vi "Playback Floor.vi"(0 "Encoder Names":string[](array[string])=["X axis", "Y axis"], 1 "Floor Recording Data":T2={"X Axis Recording Data"=[{"Encoder Position"=0.0, "Timestamp"=21}, {"Encoder Position"=0.0, "Timestamp"=41}, {"Encoder Position"=0.0, "Timestamp"=62}, {"Encoder Position"=0.0, "Timestamp"=82}, {"Encoder Position"=0.25, "Timestamp"=102}, {"Encoder Position"=0.25, "Timestamp"=122}, {"Encoder Position"=0.25, "Timestamp"=143}, {"Encoder Position"=0.25, "Timestamp"=162}, {"Encoder Position"=0.25, "Timestamp"=182}, {"Encoder Position"=0.25, "Timestamp"=202}, {"Encoder Position"=0.25, "Timestamp"=222}, {"Encoder Position"=0.75, "Timestamp"=242}, {"Encoder Position"=1.5, "Timestamp"=262}, {"Encoder Position"=2.25, "Timestamp"=282}, {"Encoder Position"=3.0, "Timestamp"=302}, {"Encoder Position"=3.75, "Timestamp"=323}, {"Encoder Position"=4.75, "Timestamp"=342}, {"Encoder Position"=5.25, "Timestamp"=363}, {"Encoder Position"=5.75, "Timestamp"=382}, {"Encoder Position"=6.5, "Timestamp"=402}, {"Encoder Position"=7.0, "Timestamp"=422}, {"Encoder Position"=7.5, "Timestamp"=443}, {"Encoder Position"=8.0, "Timestamp"=462}, {"Encoder Position"=8.25, "Timestamp"=482}, {"Encoder Position"=8.75, "Timestamp"=502}, {"Encoder Position"=8.75, "Timestamp"=522}, {"Encoder Position"=9.25, "Timestamp"=542}, {"Encoder Position"=9.25, "Timestamp"=562}, {"Encoder Position"=9.5, "Timestamp"=582}, {"Encoder Position"=9.75, "Timestamp"=602}, {"Encoder Position"=9.75, "Timestamp"=622}, {"Encoder Position"=9.75, "Timestamp"=642}, {"Encoder Position"=9.75, "Timestamp"=662}, {"Encoder Position"=9.75, "Timestamp"=683}, {"Encoder Position"=9.75, "Timestamp"=702}, {"Encoder Position"=9.75, "Timestamp"=722}, {"Encoder Position"=9.75, "Timestamp"=743}, {"Encoder Position"=10.0, "Timestamp"=763}, {"Encoder Position"=10.0, "Timestamp"=784}, {"Encoder Position"=10.25, "Timestamp"=803}, {"Encoder Position"=10.25, "Timestamp"=824}, {"Encoder Position"=10.75, "Timestamp"=844}, {"Encoder Position"=11.0, "Timestamp"=864}, {"Encoder Position"=11.5, "Timestamp"=884}, {"Encoder Position"=12.25, "Timestamp"=904}, {"Encoder Position"=13.25, "Timestamp"=924}, {"Encoder Position"=14.25, "Timestamp"=944}, {"Encoder Position"=15.75, "Timestamp"=964}, {"Encoder Position"=17.25, "Timestamp"=984}, {"Encoder Position"=18.25, "Timestamp"=1004}, {"Encoder Position"=20.25, "Timestamp"=1024}, {"Encoder Position"=22.0, "Timestamp"=1044}, {"Encoder Position"=23.75, "Timestamp"=1064}, {"Encoder Position"=26.25, "Timestamp"=1084}, {"Encoder Position"=28.75, "Timestamp"=1105}, {"Encoder Position"=30.75, "Timestamp"=1124}, {"Encoder Position"=33.0, "Timestamp"=1144}, {"Encoder Position"=35.75, "Timestamp"=1166}, {"Encoder Position"=38.75, "Timestamp"=1187}, {"Encoder Position"=42.0, "Timestamp"=1210}, {"Encoder Position"=44.25, "Timestamp"=1230}, {"Encoder Position"=47.5, "Timestamp"=1249}, {"Encoder Position"=50.25, "Timestamp"=1270}, {"Encoder Position"=53.75, "Timestamp"=1289}, {"Encoder Position"=56.75, "Timestamp"=1310}, {"Encoder Position"=59.75, "Timestamp"=1329}, {"Encoder Position"=63.0, "Timestamp"=1351}, {"Encoder Position"=66.25, "Timestamp"=1370}, {"Encoder Position"=69.5, "Timestamp"=1391}, {"Encoder Position"=72.75, "Timestamp"=1413}, {"Encoder Position"=75.5, "Timestamp"=1430}, {"Encoder Position"=78.5, "Timestamp"=1449}, {"Encoder Position"=81.75, "Timestamp"=1471}, {"Encoder Position"=85.0, "Timestamp"=1491}, {"Encoder Position"=87.75, "Timestamp"=1510}, {"Encoder Position"=90.75, "Timestamp"=1531}, {"Encoder Position"=94.25, "Timestamp"=1552}, {"Encoder Position"=96.25, "Timestamp"=1572}, {"Encoder Position"=99.75, "Timestamp"=1592}, {"Encoder Position"=102.25, "Timestamp"=1612}, {"Encoder Position"=105.0, "Timestamp"=1632}, {"Encoder Position"=107.5, "Timestamp"=1655}, {"Encoder Position"=110.0, "Timestamp"=1676}, {"Encoder Position"=112.0, "Timestamp"=1696}, {"Encoder Position"=114.25, "Timestamp"=1718}, {"Encoder Position"=116.25, "Timestamp"=1738}, {"Encoder Position"=118.0, "Timestamp"=1759}, {"Encoder Position"=119.25, "Timestamp"=1778}, {"Encoder Position"=120.25, "Timestamp"=1799}, {"Encoder Position"=120.75, "Timestamp"=1819}, {"Encoder Position"=121.75, "Timestamp"=1840}, {"Encoder Position"=122.25, "Timestamp"=1859}, {"Encoder Position"=122.75, "Timestamp"=1880}, {"Encoder Position"=122.75, "Timestamp"=1900}, {"Encoder Position"=122.75, "Timestamp"=1920}, {"Encoder Position"=122.75, "Timestamp"=1940}, {"Encoder Position"=122.75, "Timestamp"=1960}, {"Encoder Position"=122.75, "Timestamp"=1980}, {"Encoder Position"=122.75, "Timestamp"=2000}, {"Encoder Position"=122.75, "Timestamp"=2020}, {"Encoder Position"=122.75, "Timestamp"=2039}, {"Encoder Position"=122.75, "Timestamp"=2059}, {"Encoder Position"=122.75, "Timestamp"=2082}, {"Encoder Position"=122.75, "Timestamp"=2100}, {"Encoder Position"=122.75, "Timestamp"=2120}, {"Encoder Position"=122.75, "Timestamp"=2139}, {"Encoder Position"=122.75, "Timestamp"=2159}, {"Encoder Position"=122.75, "Timestamp"=2179}, {"Encoder Position"=122.75, "Timestamp"=2199}, {"Encoder Position"=122.75, "Timestamp"=2221}, {"Encoder Position"=122.75, "Timestamp"=2239}, {"Encoder Position"=122.75, "Timestamp"=2261}, {"Encoder Position"=122.75, "Timestamp"=2282}, {"Encoder Position"=122.75, "Timestamp"=2301}, {"Encoder Position"=122.75, "Timestamp"=2323}, {"Encoder Position"=122.75, "Timestamp"=2344}, {"Encoder Position"=122.75, "Timestamp"=2364}, {"Encoder Position"=122.75, "Timestamp"=2383}, {"Encoder Position"=122.75, "Timestamp"=2403}, {"Encoder Position"=122.75, "Timestamp"=2423}], "Y Axis Recording Data"=[{"Encoder Position"=0.0, "Timestamp"=21}, {"Encoder Position"=0.0, "Timestamp"=41}, {"Encoder Position"=0.0, "Timestamp"=62}, {"Encoder Position"=0.0, "Timestamp"=82}, {"Encoder Position"=0.0, "Timestamp"=102}, {"Encoder Position"=-0.25, "Timestamp"=122}, {"Encoder Position"=-0.5, "Timestamp"=143}, {"Encoder Position"=-0.75, "Timestamp"=162}, {"Encoder Position"=-1.0, "Timestamp"=182}, {"Encoder Position"=-1.5, "Timestamp"=202}, {"Encoder Position"=-2.0, "Timestamp"=222}, {"Encoder Position"=-2.5, "Timestamp"=242}, {"Encoder Position"=-3.0, "Timestamp"=262}, {"Encoder Position"=-3.5, "Timestamp"=282}, {"Encoder Position"=-4.0, "Timestamp"=302}, {"Encoder Position"=-4.5, "Timestamp"=323}, {"Encoder Position"=-5.0, "Timestamp"=342}, {"Encoder Position"=-5.5, "Timestamp"=362}, {"Encoder Position"=-6.0, "Timestamp"=383}, {"Encoder Position"=-6.5, "Timestamp"=402}, {"Encoder Position"=-7.0, "Timestamp"=422}, {"Encoder Position"=-7.5, "Timestamp"=443}, {"Encoder Position"=-8.0, "Timestamp"=462}, {"Encoder Position"=-8.5, "Timestamp"=482}, {"Encoder Position"=-9.0, "Timestamp"=502}, {"Encoder Position"=-9.5, "Timestamp"=522}, {"Encoder Position"=-9.75, "Timestamp"=542}, {"Encoder Position"=-10.25, "Timestamp"=562}, {"Encoder Position"=-10.5, "Timestamp"=582}, {"Encoder Position"=-10.75, "Timestamp"=602}, {"Encoder Position"=-11.0, "Timestamp"=622}, {"Encoder Position"=-11.25, "Timestamp"=642}, {"Encoder Position"=-11.25, "Timestamp"=662}, {"Encoder Position"=-11.5, "Timestamp"=683}, {"Encoder Position"=-11.5, "Timestamp"=702}, {"Encoder Position"=-11.5, "Timestamp"=722}, {"Encoder Position"=-11.5, "Timestamp"=743}, {"Encoder Position"=-11.25, "Timestamp"=763}, {"Encoder Position"=-11.25, "Timestamp"=784}, {"Encoder Position"=-11.25, "Timestamp"=803}, {"Encoder Position"=-11.25, "Timestamp"=824}, {"Encoder Position"=-11.25, "Timestamp"=844}, {"Encoder Position"=-11.25, "Timestamp"=864}, {"Encoder Position"=-11.25, "Timestamp"=884}, {"Encoder Position"=-11.0, "Timestamp"=904}, {"Encoder Position"=-11.0, "Timestamp"=924}, {"Encoder Position"=-10.75, "Timestamp"=944}, {"Encoder Position"=-10.5, "Timestamp"=964}, {"Encoder Position"=-10.5, "Timestamp"=984}, {"Encoder Position"=-10.5, "Timestamp"=1004}, {"Encoder Position"=-10.5, "Timestamp"=1024}, {"Encoder Position"=-10.5, "Timestamp"=1044}, {"Encoder Position"=-10.5, "Timestamp"=1064}, {"Encoder Position"=-10.5, "Timestamp"=1084}, {"Encoder Position"=-10.5, "Timestamp"=1105}, {"Encoder Position"=-10.5, "Timestamp"=1124}, {"Encoder Position"=-10.5, "Timestamp"=1144}, {"Encoder Position"=-10.5, "Timestamp"=1167}, {"Encoder Position"=-10.5, "Timestamp"=1187}, {"Encoder Position"=-10.5, "Timestamp"=1209}, {"Encoder Position"=-10.5, "Timestamp"=1230}, {"Encoder Position"=-10.5, "Timestamp"=1249}, {"Encoder Position"=-10.5, "Timestamp"=1270}, {"Encoder Position"=-10.5, "Timestamp"=1289}, {"Encoder Position"=-10.5, "Timestamp"=1309}, {"Encoder Position"=-10.5, "Timestamp"=1329}, {"Encoder Position"=-10.5, "Timestamp"=1350}, {"Encoder Position"=-10.5, "Timestamp"=1370}, {"Encoder Position"=-10.5, "Timestamp"=1391}, {"Encoder Position"=-10.5, "Timestamp"=1413}, {"Encoder Position"=-10.5, "Timestamp"=1430}, {"Encoder Position"=-10.5, "Timestamp"=1449}, {"Encoder Position"=-10.5, "Timestamp"=1470}, {"Encoder Position"=-10.5, "Timestamp"=1491}, {"Encoder Position"=-10.25, "Timestamp"=1510}, {"Encoder Position"=-10.0, "Timestamp"=1531}, {"Encoder Position"=-9.75, "Timestamp"=1552}, {"Encoder Position"=-9.75, "Timestamp"=1572}, {"Encoder Position"=-9.5, "Timestamp"=1592}, {"Encoder Position"=-9.25, "Timestamp"=1612}, {"Encoder Position"=-9.0, "Timestamp"=1633}, {"Encoder Position"=-8.5, "Timestamp"=1655}, {"Encoder Position"=-8.5, "Timestamp"=1675}, {"Encoder Position"=-8.0, "Timestamp"=1695}, {"Encoder Position"=-8.0, "Timestamp"=1718}, {"Encoder Position"=-7.75, "Timestamp"=1738}, {"Encoder Position"=-7.5, "Timestamp"=1759}, {"Encoder Position"=-7.25, "Timestamp"=1778}, {"Encoder Position"=-7.0, "Timestamp"=1799}, {"Encoder Position"=-6.75, "Timestamp"=1819}, {"Encoder Position"=-6.5, "Timestamp"=1840}, {"Encoder Position"=-6.5, "Timestamp"=1859}, {"Encoder Position"=-6.0, "Timestamp"=1880}, {"Encoder Position"=-5.75, "Timestamp"=1900}, {"Encoder Position"=-5.5, "Timestamp"=1920}, {"Encoder Position"=-5.5, "Timestamp"=1940}, {"Encoder Position"=-5.25, "Timestamp"=1960}, {"Encoder Position"=-5.0, "Timestamp"=1979}, {"Encoder Position"=-5.0, "Timestamp"=2001}, {"Encoder Position"=-5.0, "Timestamp"=2020}, {"Encoder Position"=-4.75, "Timestamp"=2040}, {"Encoder Position"=-4.75, "Timestamp"=2059}, {"Encoder Position"=-4.75, "Timestamp"=2082}, {"Encoder Position"=-4.75, "Timestamp"=2100}, {"Encoder Position"=-4.75, "Timestamp"=2120}, {"Encoder Position"=-4.75, "Timestamp"=2139}, {"Encoder Position"=-4.75, "Timestamp"=2159}, {"Encoder Position"=-4.75, "Timestamp"=2182}, {"Encoder Position"=-4.75, "Timestamp"=2199}, {"Encoder Position"=-4.75, "Timestamp"=2221}, {"Encoder Position"=-4.75, "Timestamp"=2239}, {"Encoder Position"=-4.75, "Timestamp"=2261}, {"Encoder Position"=-4.75, "Timestamp"=2282}, {"Encoder Position"=-4.75, "Timestamp"=2302}, {"Encoder Position"=-4.75, "Timestamp"=2323}, {"Encoder Position"=-4.75, "Timestamp"=2344}, {"Encoder Position"=-4.75, "Timestamp"=2364}, {"Encoder Position"=-4.75, "Timestamp"=2383}, {"Encoder Position"=-4.75, "Timestamp"=2404}, {"Encoder Position"=-4.75, "Timestamp"=2424}]}, 2 "Playback allow":bool=TRUE, 4 "Playback":bool=TRUE, 5 "Rewind":bool, 6 "Home":bool) -> (9 "End of Playback":bool, 10 "X Encoder Distance PB":dbl=-402.0)   [LabVIEW 2017]
uses:
  <vilib>/Rock Robotics/WPI/Utilities/WPI_GetSetVariantRefNum.vi
  <vilib>/addons/control/pid/pid.llb/PID (DBL).vi
  <vilib>/Rock Robotics/WPI/RobotDrive/WPI_RobotDriveMecanumDrive_Cartesian.vi
  <vilib>/addons/control/pid/NI_PID_pid.lvlib
panel:
  in  "Motor Name":string="Four Motors"
  in  "Y Playback PID gains":T1={"proportional gain (Kc)"=-0.004, "integral time (Ti, min)"=0.0, "derivative time (Td, min)"=0.0} {"derivative time (Td, min)" format="%.8f"; "integral time (Ti, min)" format="%.8f"; "proportional gain (Kc)" format="%.8f"}
  out "Y Initial Encoder Position":dbl=138.25
  out "Y Encoder Distance PB":dbl=148.0
  out "X Initial Encoder Position":dbl=-139.5
  in  "Taper Limit":dbl=1.0
  out "Waveform Chart":T3(graph)={"Encoder Position"=122.75, -262.5, "Encoder Position"=-5.0, 9.75}
  in  "X Playback PID gains":T1={"proportional gain (Kc)"=-0.008, "integral time (Ti, min)"=0.0, "derivative time (Td, min)"=0.0} {"derivative time (Td, min)" format="%.8f"; "integral time (Ti, min)" format="%.8f"; "proportional gain (Kc)" format="%.8f"}
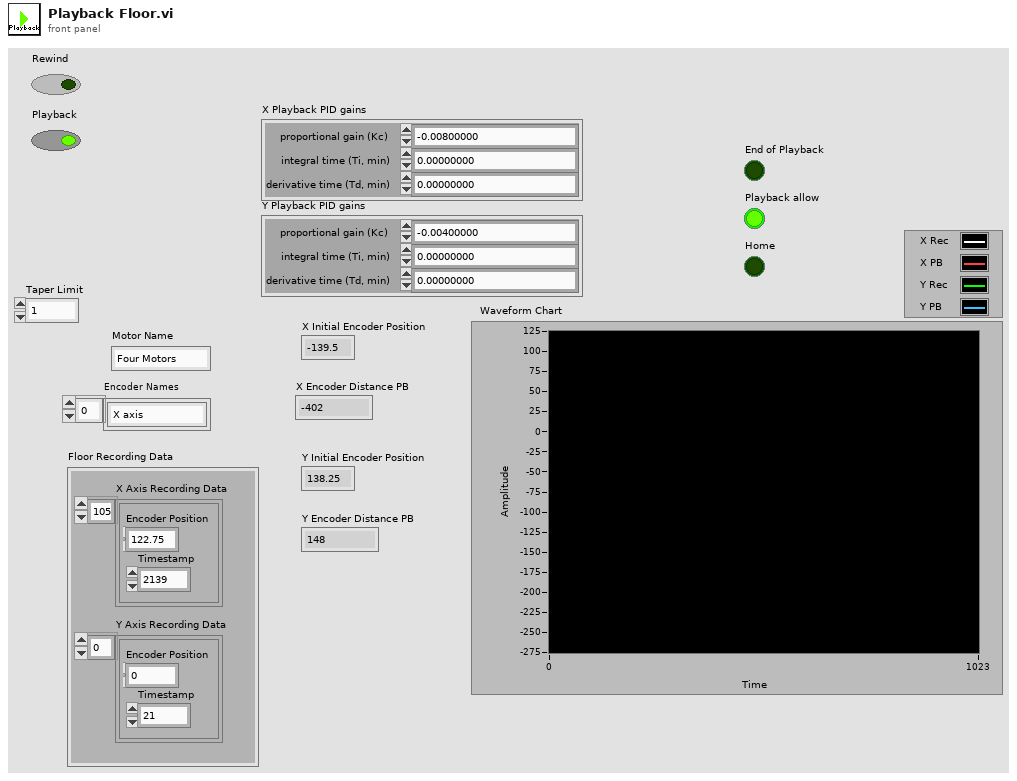
[diagram p1: front panel]
types:
  T1 = cluster{"proportional gain (Kc)":dbl, "integral time (Ti, min)":dbl, "derivative time (Td, min)":dbl}
  T2 = cluster{"X Axis Recording Data":cluster{"Encoder Position":dbl, "Timestamp":i32}[], "Y Axis Recording Data":cluster{"Encoder Position":dbl, "Timestamp":i32}[]}
  T3 = cluster{"Encoder Position":dbl, dbl, "Encoder Position":dbl, dbl}
  T4 = cluster{"Encoder Position":dbl, "Timestamp":i32}[]
  T5 = typedef "WPI_RobotDriveDevRef.ctl" = cluster{"DevStatus":errorcluster, "Motors[]":T6[], "Square Inputs":bool, "Max Output":dbl}
  T6 = typedef "WPI_MotorControlDeviceRef.ctl" = cluster{"DeviceStatus":errorcluster, "Type":T7, "PWM":cluster{"PWM Channel":T8, "DeadBand":T9}, "CAN":cluster{"Device Number":u8, "SetOutput VI Ref":variant, "GetOutput VI Ref":variant, "Enable VI Ref":variant, "Disable VI Ref":variant, "Data":variant}, "Invert":bool, "DIO PWM":cluster{"PWM \"Enable\" Channel":T8, "DIOChannel":T10, "PWM Rate":dbl}}
  T7 = typedef "WPI_MotorControlType.ctl" = enum16{"PWM", "CAN", "DIO PWM"}
  T8 = typedef "FPGA_DIOPWMChannel.ctl" = enum8{"PWM 0", "PWM 1", "PWM 2", "PWM 3", "PWM 4", "PWM 5", "PWM 6", "PWM 7", "PWM 8", "PWM 9", "PWM MXP 0", "PWM MXP 1", "PWM MXP 2", "PWM MXP 3", "PWM MXP 4", "PWM MXP 5", "PWM MXP 6", "PWM MXP 7", "PWM MXP 8", "PWM MXP 9", "Invalid"}
  T9 = typedef "WPI_PWMDeadband.ctl" = cluster{"Name":string, "maxPositivePwm":i32, "minPositivePwm":i32, "centerPwm":i32, "maxNegativePwm":i32, "minNegativePwm":i32, "angularRange":u16}
  T10 = typedef "FPGA_DIOChannel.ctl" = enum8{"DIO 0", "DIO 1", "DIO 2", "DIO 3", "DIO 4", "DIO 5", "DIO 6", "DIO 7", "DIO 8", "DIO 9", "DIO MXP 0", "DIO MXP 1", "DIO MXP 2", "DIO MXP 3", "DIO MXP 4", "DIO MXP 5", "DIO MXP 6", "DIO MXP 7", "DIO MXP 8", "DIO MXP 9", "DIO MXP 10", "DIO MXP 11", "DIO MXP 12", "DIO MXP 13", "DIO MXP 14", "DIO MXP 15", "SPI Port CS1", "SPI Port CS2", "SPI Port CS3", "SPI Port MISO", "SPI Port MOSI", "Invalid"}
  T11 = typedef "WPI_EncoderDevRef.ctl" = cluster{"DevStatus":errorcluster, "EncoderIndex":T12, "CounterIndex":T13, "DistancePerCount":dbl, "Decoding Type":T14}
  T12 = typedef "FPGA_EncoderIdx.ctl" = enum8{"Enc 0", "Enc 1", "Enc 2", "Enc 3", "Enc 4", "Enc 5", "Enc 6", "Enc 7", "Invalid"}
  T13 = typedef "FPGA_CounterCtrSystemIndex.ctl" = enum8{"Ctr 0", "Ctr 1", "Ctr 2", "Ctr 3", "Ctr 4", "Ctr 5", "Ctr 6", "Ctr 7", "Invalid"}
  T14 = typedef "WPI_EncoderType.ctl" = enum16{"1x", "2x", "4x"}
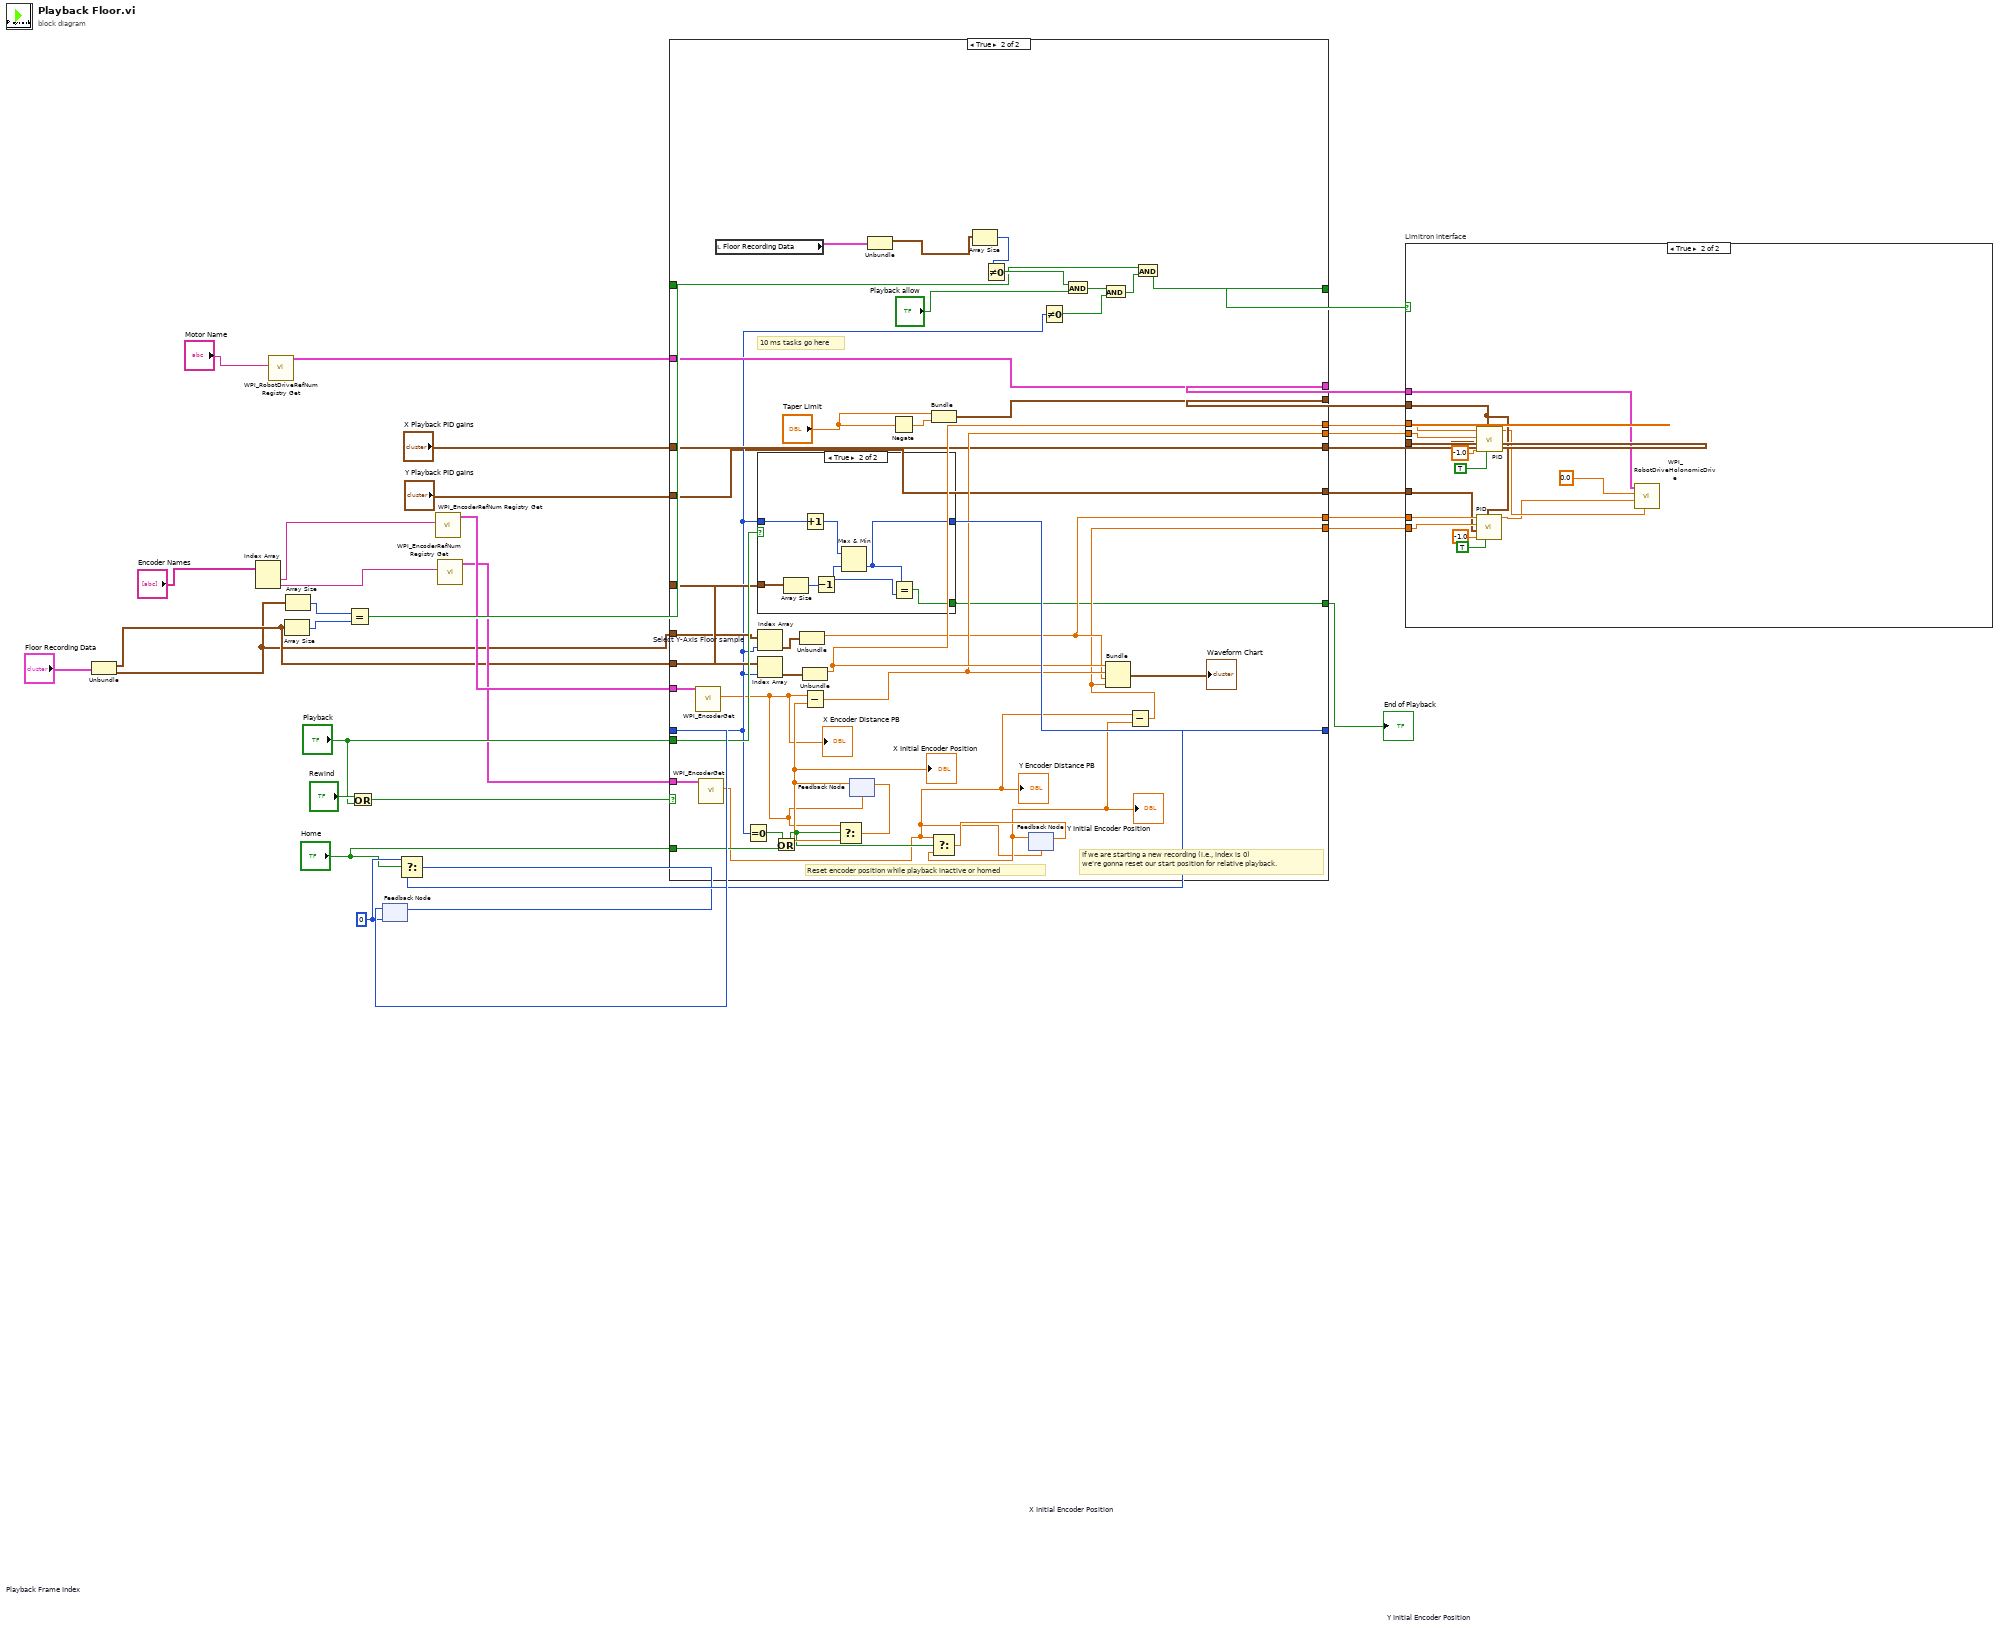
[diagram p0: block diagram]
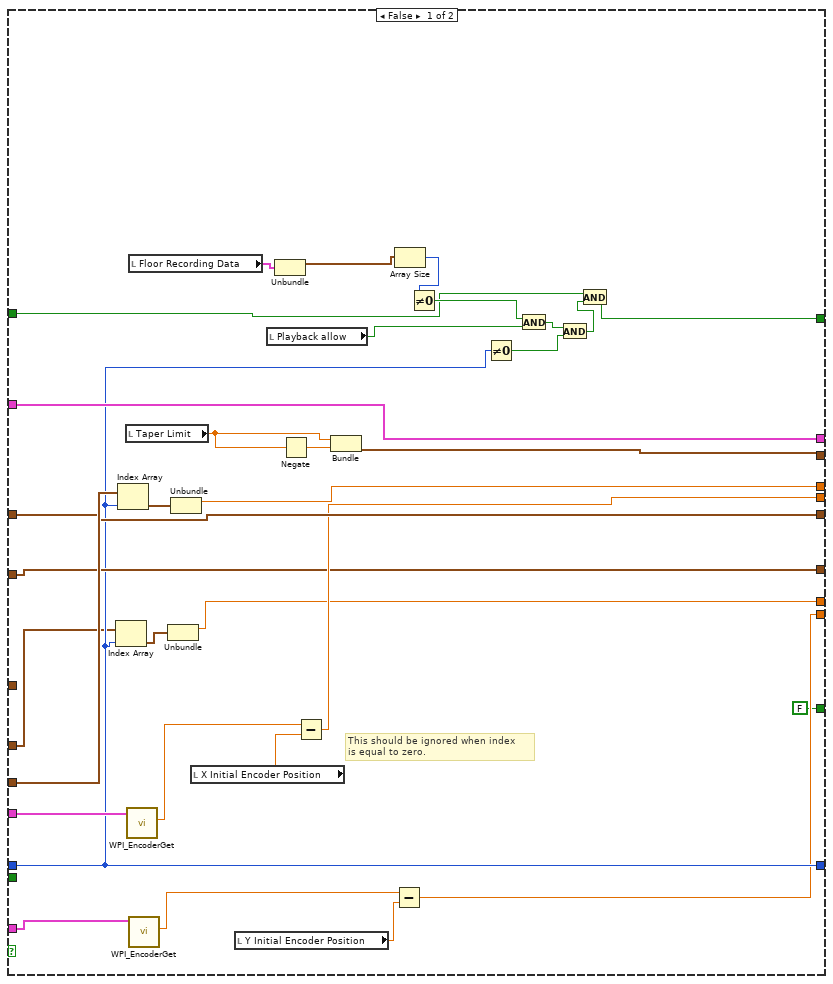
[diagram p3: hidden frame]
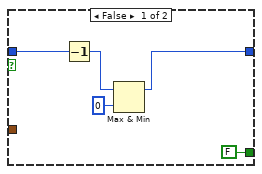
[diagram p4: hidden frame]
diagram:
  w26 = 0 ("index")
  n1 = Unbundle("Floor Recording Data") -> ("X Axis Recording Data"=w8:T4, "Y Axis Recording Data"=w7:T4)
  n2 = Index Array(array="Encoder Names") -> (element #1=w12:string, element #2=w10:string)  [unwired: 2 in]
  n3 = call <vilib>:"WPI_RobotDriveRefNum Registry Get.vi"("refnum name"="Motor Name") -> ("RobotDriveDevRef"=w33:T5)  [unwired: 1 in, 9 out]
  n4 = Array Size(array=w8) -> (size(s)=w16:i32)
  n5 = Array Size(array=w7) -> (size(s)=w15:i32)
  n6 = Equal?(x=w15, y=w16) -> (x = y?=w14:bool)
  n7 = Or(x="Rewind", y="Playback") -> (x .or. y?=w31:bool)
  n8 = feedback #1 "Playback Frame Index"(w26) -> (w29:i32)
  n9 = call <vilib>:"WPI_EncoderRefNum Registry Get.vi"("refnum name"=w12) -> ("EncoderDevRef"=w11:T11)  [unwired: 9 in, 1 out]
  n10 = call <vilib>:"WPI_EncoderRefNum Registry Get.vi"("refnum name"=w10) -> ("EncoderDevRef"=w9:T11)  [unwired: 9 in, 1 out]
  n11 = case shown="True" w31 {
    tunnel: w11 -> [w54 w75]
    tunnel: w33 -> [w61 w97]
    tunnel: "Playback" -> [_ w106]
    tunnel: w8 -> [w65 w101]
    tunnel: w29 -> [w42 w78]
    tunnel: [w42 w100] -> w27
    tunnel: "X Playback PID gains" -> [w59 w93]
    tunnel: w8 -> [_ w98]
    tunnel: [w61 w97] -> w24
    tunnel: [w60 w96] -> w23
    tunnel: [w51 w95] -> w22
    tunnel: [w58 w94] -> w21
    tunnel: [w59 w93] -> w20
    tunnel: [w46 w82] -> w19
    tunnel: "Home" -> [_ w85]
    tunnel: w14 -> [w47 w83]
    tunnel: w7 -> [w41 w79]
    tunnel: w9 -> [w38 w73]
    tunnel: [w39 w69] -> w6
    tunnel: [w35 w68] -> w5
    tunnel: [w43 w67] -> w4
    tunnel: "Y Playback PID gains" -> [w43 w67]
    tunnel: [FALSE w66] -> w1
    frame False {
      # "This should be ignored when index \nis equal to zero."
      n12 = Index Array(array=w41, index=w42) -> (element=w40:cluster{"Encoder Position":dbl, "Timestamp":i32})
      n13 = Index Array(array=w65, index=w42) -> (element=w64:cluster{"Encoder Position":dbl, "Timestamp":i32})
      n14 = local read "Taper Limit"() -> (w62:dbl)
      n15 = call <vilib>:"WPI_EncoderGet.vi"("EncoderDevRef"=w54) -> ("Distance"=w53:dbl)  [unwired: 5 in, 5 out]
      n16 = local read "Floor Recording Data"() -> (w45:T2)
      n17 = call <vilib>:"WPI_EncoderGet.vi"("EncoderDevRef"=w38) -> ("Distance"=w37:dbl)  [unwired: 5 in, 5 out]
      n18 = Unbundle(w40) -> ("Encoder Position"=w39:dbl)  [unwired: 1 out]
      n19 = Unbundle(w64) -> ("Encoder Position"=w60:dbl)  [unwired: 1 out]
      n20 = local read "X Initial Encoder Position"() -> (w52:dbl)
      n21 = local read "Y Initial Encoder Position"() -> (w36:dbl)
      n22 = local read "Playback allow"() -> (w55:bool)
      n23 = Unbundle(w45) -> ("X Axis Recording Data"=w44:T4)  [unwired: 1 out]
      n24 = Negate(x=w62) -> (-x=w63:dbl)
      n25 = Subtract(x=w53, y=w52) -> (x-y=w51:dbl)
      n26 = Bundle("Taper Limit"=w62, w63) -> (w58:cluster{"Taper Limit":dbl, dbl})  [unwired: 1 in]
      n27 = Subtract(x=w37, y=w36) -> (x-y=w35:dbl)
      n28 = Array Size(array=w44) -> (size(s)=w57:i32)
      n29 = Not Equal To 0?(x=w57) -> (x != 0?=w56:bool)
      n30 = Not Equal To 0?(x=w42) -> (x != 0?=w49:bool)
      n31 = And(x=w56, y=w55) -> (x .and. y?=w50:bool)
      n32 = And(x=w50, y=w49) -> (x .and. y?=w48:bool)
      n33 = And(x=w47, y=w48) -> (x .and. y?=w46:bool)
    }
    frame True {
      # "Reset encoder position while playback inactive or homed"
      # "If we are starting a new recording (i.e., index is 0)\nwe're gonna reset our start position for relative playback."
      # "10 ms tasks go here"
      n34 = call <vilib>:"WPI_EncoderGet.vi"("EncoderDevRef"=w75) -> ("Distance"=w76:dbl)  [unwired: 5 in, 5 out]
      "X Encoder Distance PB" <- w76
      n35 = call <vilib>:"WPI_EncoderGet.vi"("EncoderDevRef"=w73) -> ("Distance"=w70:dbl)  [unwired: 5 in, 5 out]
      "Y Encoder Distance PB" <- w70
      n36 = local read "Floor Recording Data"() -> (w81:T2)
      n37 = Equal To 0?(x=w78) -> (x = 0?=w86:bool)
      n38 = case shown="True" w106 {
        tunnel: [w108 w113] -> w100
        tunnel: w78 -> [w111 w118]
        tunnel: w98 -> [_ w116]
        tunnel: [FALSE w112] -> w66
        frame False {
          n39 = Decrement(x=w111) -> (x-1=w109:i32)
          n40 = Max & Min(x=w109, y=0) -> (max(x,y)=w108:i32)  [unwired: 1 out]
        }
        frame True {
          n41 = Array Size(array=w116) -> (size(s)=w115:i32)
          n42 = Increment(x=w118) -> (x+1=w117:i32)
          n43 = Decrement(x=w115) -> (x-1=w114:i32)
          n44 = Max & Min(x=w117, y=w114) -> (min(x,y)=w113:i32)  [unwired: 1 out]
          n45 = Equal?(x=w113, y=w114) -> (x = y?=w112:bool)
        }
      }
      n46 = Index Array "Select Y-Axis Floor sample"(array=w79, index=w78) -> (element=w77:cluster{"Encoder Position":dbl, "Timestamp":i32})
      n47 = Index Array(array=w101, index=w78) -> (element=w102:cluster{"Encoder Position":dbl, "Timestamp":i32})
      n48 = Or(x=w86, y=w85) -> (x .or. y?=w74:bool)
      n49 = Unbundle(w77) -> ("Encoder Position"=w69:dbl)  [unwired: 1 out]
      n50 = Unbundle(w102) -> ("Encoder Position"=w96:dbl)  [unwired: 1 out]
      n51 = feedback #2 "X Initial Encoder Position"(w76) -> (w99:dbl)
      "X Initial Encoder Position" <- w99
      n52 = Subtract(x=w76, y=w99) -> (x-y=w95:dbl)
      n53 = Select(t=w76, s=w74, f=w99) -> (s? t:f=w89:dbl)
      n54 = feedback-in #2(w89) -> ()
      n55 = Unbundle(w81) -> ("X Axis Recording Data"=w80:T4)  [unwired: 1 out]
      n56 = Negate(x="Taper Limit") -> (-x=w104:dbl)
      n57 = Bundle("Taper Limit"="Taper Limit", w104) -> (w94:cluster{"Taper Limit":dbl, dbl})  [unwired: 1 in]
      n58 = Array Size(array=w80) -> (size(s)=w92:i32)
      n59 = Not Equal To 0?(x=w92) -> (x != 0?=w90:bool)
      n60 = feedback #3 "Y Initial Encoder Position"(w70) -> (w71:dbl)
      "Y Initial Encoder Position" <- w71
      n61 = Select(t=w70, s=w74, f=w71) -> (s? t:f=w72:dbl)
      n62 = feedback-in #3(w72) -> ()
      n63 = Not Equal To 0?(x=w78) -> (x != 0?=w87:bool)
      n64 = And(x=w90, y="Playback allow") -> (x .and. y?=w88:bool)
      n65 = And(x=w88, y=w87) -> (x .and. y?=w84:bool)
      n66 = Subtract(x=w70, y=w71) -> (x-y=w68:dbl)
      n67 = Bundle("Encoder Position"=w96, w95, "Encoder Position"=w69, w68) -> (→"Waveform Chart":T3)  [unwired: 1 in]
      n68 = And(x=w83, y=w84) -> (x .and. y?=w82:bool)
    }
  }
  "End of Playback" <- w1
  n69 = Select(t=w26, s="Home", f=w27) -> (s? t:f=w25:i32)
  n70 = feedback-in #1(w25) -> ()
  n71 = case "Limitron interface" shown="True" w19 {
    tunnel: w20 -> [_ w133]
    tunnel: w22 -> [_ w130]
    tunnel: w23 -> [_ w129]
    tunnel: w24 -> [_ w122]
    tunnel: w21 -> [_ w124]
    tunnel: w6 -> [_ w127]
    tunnel: w5 -> [_ w126]
    tunnel: w4 -> [_ w125]
    frame False {
    }
    frame True {
      n72 = call-poly <vilib>:"PID.vi"("reinitialize? (F)"=TRUE, "output range"=w124, "dt (s)"=-1.0, "PID gains"=w125, "process variable"=w126, "setpoint"=w127) -> ("output"=w120:dbl)  [unwired: 4 in, 1 out]
      n73 = call-poly <vilib>:"PID.vi"("reinitialize? (F)"=TRUE, "output range"=w124, "dt (s)"=-1.0, "PID gains"=w133, "process variable"=w130, "setpoint"=w129) -> ("output"=w121:dbl)  [unwired: 4 in, 1 out]
      n74 = call-poly <vilib>:"WPI_RobotDriveHolonomicDrive.vi"("Rotation"=w121, "Y"=w120, "X"=0.0, "RobotDriveDevRef"=w122) -> ()  [unwired: 5 in, 3 out]
    }
  }
